vi "UI Coherent.vi"(8 "error in":errorcluster) -> (0 "error out":errorcluster)   [LabVIEW 2019, in "Coherent.lvlib"]
uses:
  Coherent.lvlib
  User Event/Controls/UE Abort Action.ctl
  <vilib>/Utility/miscctls.llb/LVPointTypeDef.ctl
  Queues/Queues.lvlib
panel:
  in  "Laser Control":T1={"Laser Switch"=FALSE, "Laser Power(mW)"=40} {"Laser Power(mW)" max=100}
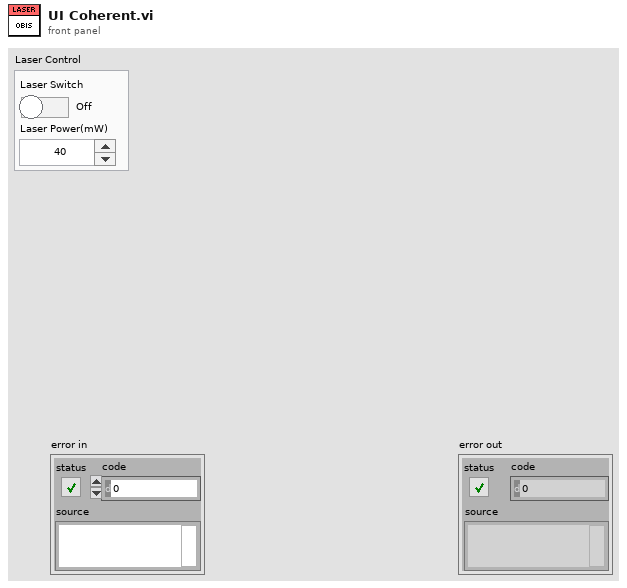
[diagram p1: front panel]
types:
  T1 = cluster{"Laser Switch":bool, "Laser Power(mW)":u16}
  T2 = typedef "UE Abort Action.ctl" = enum16{"Create", "Get", "Destroy"}
  T3 = enum16{"Start", "Get State", "On", "Off", "Set Power", "Change Mode", "Close"}
  T4 = typedef "LVPointTypeDef.ctl" = cluster{"Horizontal":i16, "Vertical":i16}
  T5 = typedef "Coherent.lvlib/SEQ Data.ctl" = cluster{"Initialize Success?":bool, "VI Refnum":refnum<vi>}
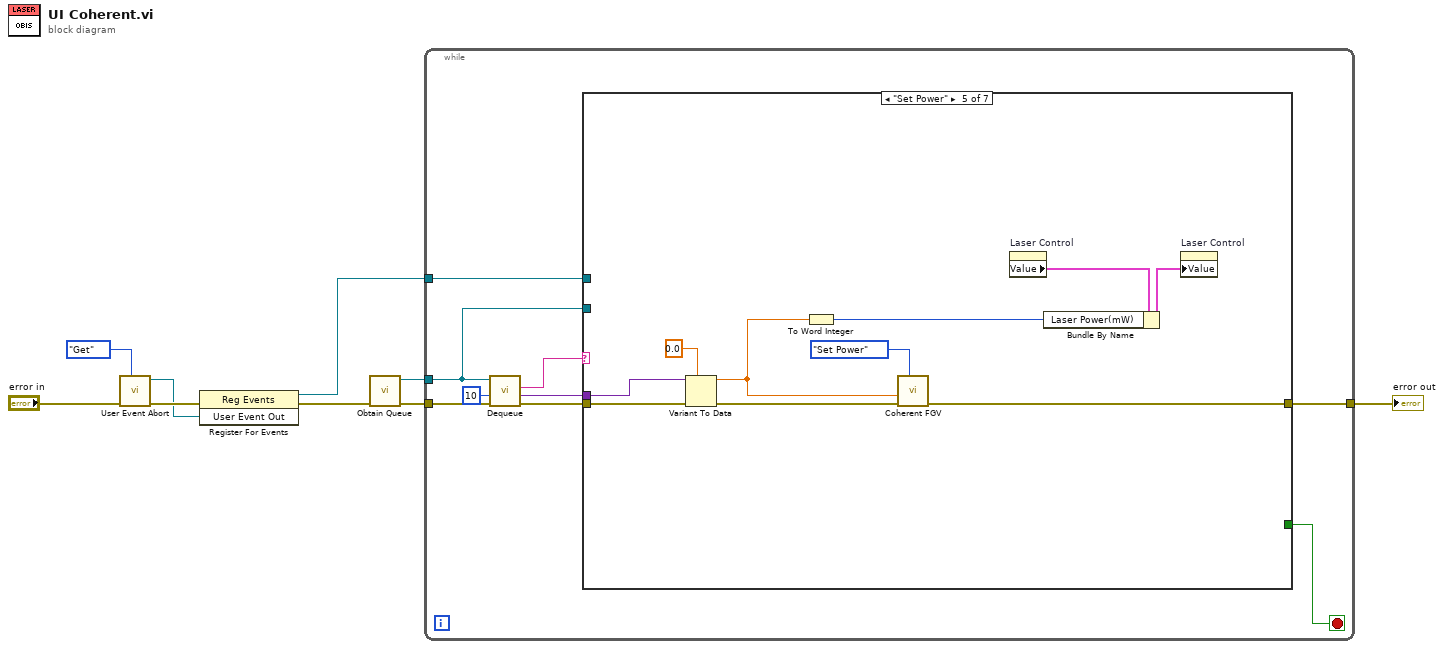
[diagram p0: block diagram]
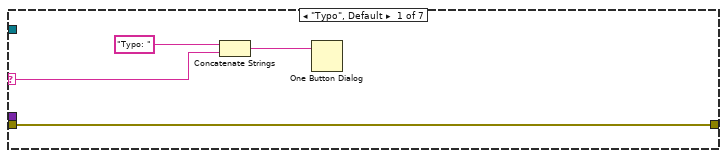
[diagram p2: hidden frame]
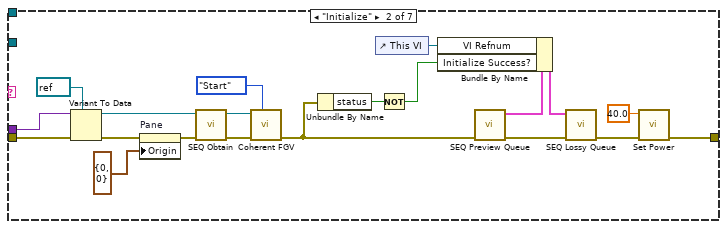
[diagram p3: hidden frame]
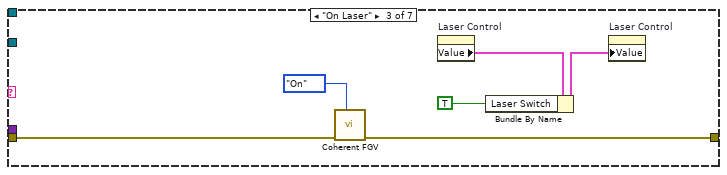
[diagram p4: hidden frame]
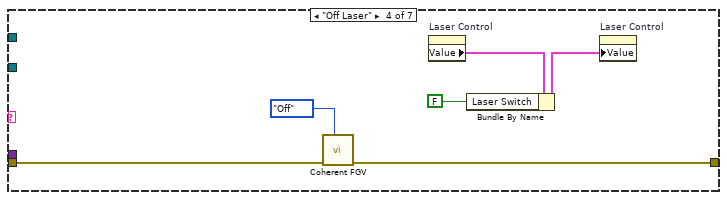
[diagram p5: hidden frame]
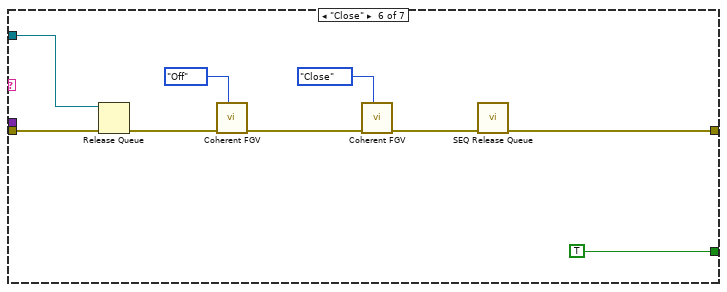
[diagram p6: hidden frame]
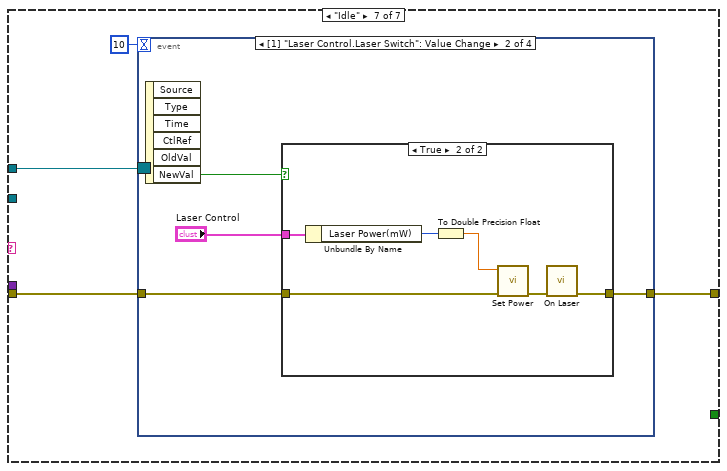
[diagram p7: hidden frame]
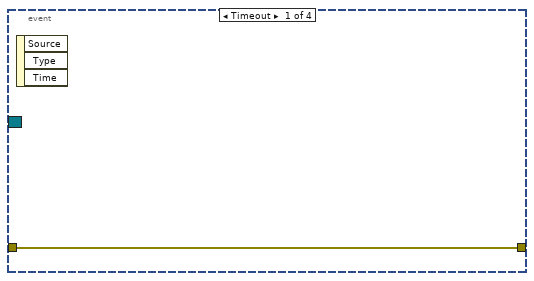
[diagram p8: hidden frame]
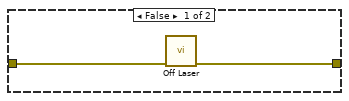
[diagram p9: hidden frame]
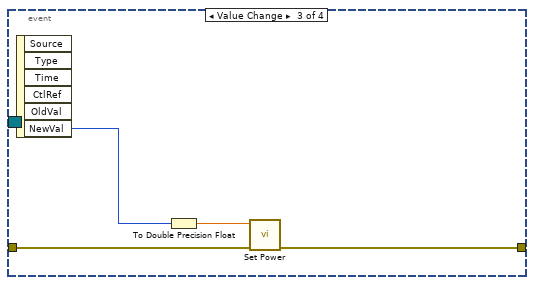
[diagram p10: hidden frame]
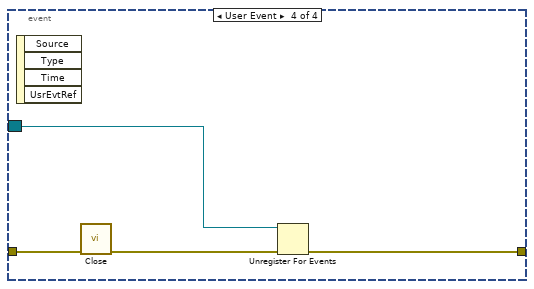
[diagram p11: hidden frame]
diagram:
  n1 = call "User Event Abort.vi"("Action"=UE_Abort_Action."Get", "Error In"="error in") -> ("Error Out"=w7:errorcluster, "User Event Out"=w6:refnum<user-event>)  [unwired: 8 in]
  n2 = register-events(error in=w7, w6) -> (reference out=w4:refnum<event-registration>, error out=w3:errorcluster)  [unwired: 1 in]
  n3 = call "Obtain Queue.vi"("Error In"=w3) -> ("Error Out"=w2:errorcluster, "Queue out"=w1:refnum<queue>)  [unwired: 9 in]
  n4 = while {
    tunnel: w2 -> [w18]
    tunnel: w1 -> [w13]
    tunnel: [w12] -> w5
    tunnel: w4 -> [w11]
    stop <- w10 stop-if-true
    n5 = call "Dequeue.vi"("Error In"=w18, "timeout in ms (-1)"=10, "Queue in"=w13) -> ("Error Out"=w17:errorcluster, "Data"=w15:variant, "State"=w16:string)  [unwired: 5 in, 1 out]
    n6 = case shown="\"Set Power\"" w16 {
      selector: w16 -> [w19 _ _ _ _ _ _]
      tunnel: w17 -> [w22 w29 w47 w53 w61 w72 w75]
      tunnel: w15 -> [_ w27 _ _ w59 _ _]
      tunnel: w13 -> [_ _ _ _ _ w71 _]
      tunnel: [w22 w39 w46 w52 w63 w67 w74] -> w12
      tunnel: w11 -> [_ _ _ _ _ _ w73]
      tunnel: [_ _ _ _ _ TRUE _] -> w10
      frame "Typo", Default {
        n7 = Concatenate Strings("Typo: " ("string"), w19) -> (w21:string)
        n8 = One Button Dialog(message=w21) -> ()  [unwired: 1 in, 1 out]
      }
      frame "Initialize" {
        n9 = Variant To Data(error in=w29, type=refnum<visa-resource-name> refnum ("VISA resource name in"), Variant=w27) -> (data=w25:refnum<visa-resource-name>, error out=w28:errorcluster)
        n10 = property on="Pane" class="Pane"(error in=w28, "Origin"=T4 {"Horizontal"=0, "Vertical"=0}) -> (error out=w40:errorcluster)  [unwired: 1 in, 1 out]
        n11 = call "SEQ Obtain.vi"("error in"=w40) -> ("error out"=w30:errorcluster)  [unwired: 9 in, 1 out]
        n12 = call "Coherent FGV.vi"("Funtion"=T3."Start", "error in"=w30, "VISA resource name in"=w25) -> ("error out"=w35:errorcluster)  [unwired: 7 in, 1 out]
        n13 = Unbundle By Name(w35) -> ("status"=w24:bool)
        n14 = control-ref of="This VI"() -> (w34:refnum<vi>)
        n15 = Not(x=w24) -> (.not. x?=w23:bool)
        n16 = call "SEQ Preview Queue.vi"("error in"=w35) -> ("error out"=w38:errorcluster, "SEQ Data"=w37:T5)  [unwired: 9 in]
        n17 = Bundle By Name(cluster=w37, "VI Refnum"=w34, "Initialize Success?"=w23) -> (w36:T5)
        n18 = call "SEQ Lossy Queue.vi"("error in"=w38, "SEQ Data"=w36) -> ("error out"=w32:errorcluster)  [unwired: 9 in]
        n19 = call "Set Power.vi"("Error In"=w32, "Power(mW)"=40.0) -> ("Error Out"=w39:errorcluster)  [unwired: 9 in]
      }
      frame "On Laser" {
        n20 = call "Coherent FGV.vi"("Funtion"=T3."On", "error in"=w47) -> ("error out"=w46:errorcluster)  [unwired: 8 in, 1 out]
        n21 = property on="Laser Control" class="Clust (strict)"() -> ("Value"=w44:T1)  [unwired: 2 in, 2 out]
        n22 = Bundle By Name(cluster=w44, "Laser Switch"=TRUE) -> (w43:T1)
        n23 = property on="Laser Control" class="Clust (strict)"("Value"=w43) -> ()  [unwired: 2 in, 2 out]
      }
      frame "Off Laser" {
        n24 = call "Coherent FGV.vi"("Funtion"=T3."Off", "error in"=w53) -> ("error out"=w52:errorcluster)  [unwired: 8 in, 1 out]
        n25 = property on="Laser Control" class="Clust (strict)"() -> ("Value"=w50:T1)  [unwired: 2 in, 2 out]
        n26 = Bundle By Name(cluster=w50, "Laser Switch"=FALSE) -> (w49:T1)
        n27 = property on="Laser Control" class="Clust (strict)"("Value"=w49) -> ()  [unwired: 2 in, 2 out]
      }
      frame "Set Power" {
        n28 = Variant To Data(error in=w61, type=0.0 ("Power(mW)"), Variant=w59) -> (data=w55:dbl, error out=w60:errorcluster)
        n29 = To Word Integer(number=w55) -> (16bit integer=w54:i16)
        n30 = call "Coherent FGV.vi"("Funtion"=T3."Set Power", "error in"=w60, "Power(mW)"=w55) -> ("error out"=w63:errorcluster)  [unwired: 7 in, 1 out]
        n31 = property on="Laser Control" class="Clust (strict)"() -> ("Value"=w57:T1)  [unwired: 2 in, 2 out]
        n32 = Bundle By Name(cluster=w57, "Laser Power(mW)"=w54) -> (w56:T1)
        n33 = property on="Laser Control" class="Clust (strict)"("Value"=w56) -> ()  [unwired: 2 in, 2 out]
      }
      frame "Close" {
        n34 = Release Queue(queue=w71, error in (no error)=w72) -> (error out=w65:errorcluster)  [unwired: 1 in, 2 out]
        n35 = call "Coherent FGV.vi"("Funtion"=T3."Off", "error in"=w65) -> ("error out"=w64:errorcluster)  [unwired: 8 in, 1 out]
        n36 = call "Coherent FGV.vi"("Funtion"=T3."Close", "error in"=w64) -> ("error out"=w68:errorcluster)  [unwired: 8 in, 1 out]
        n37 = call "SEQ Release Queue.vi"("error in"=w68) -> ("error out"=w67:errorcluster)  [unwired: 10 in]
      }
      frame "Idle" {
        n38 = event shown="[1] \"Laser Control.Laser Switch\": Value Change" {
          selector: w73 -> [_ _ _ w97]
          dyn-events: _ -> [_ _ _ _]
          timeout: 10 -> [_ _ _ _]
          tunnel: w75 -> [w77 w80 w93 w95]
          tunnel: [w77 w79 w92 w96] -> w74
          event Timeout {
            n39 = event-data() -> ()  [unwired: 1 in, 3 out]
          }
          event "Laser Control.Laser Switch": Value Change {
            n40 = event-data() -> ("NewVal"=w81:bool)  [unwired: 1 in, 5 out]
            n41 = case shown="True" w81 {
              tunnel: w80 -> [w83 w86]
              tunnel: [w82 w89] -> w79
              tunnel: "Laser Control" -> [_ w88]
              frame False {
                n42 = call "Off Laser.vi"("Error In"=w83) -> ("Error Out"=w82:errorcluster)  [unwired: 10 in]
              }
              frame True {
                n43 = Unbundle By Name(w88) -> ("Laser Power(mW)"=w87:u16)
                n44 = To Double Precision Float(number=w87) -> (double precision float=w84:dbl)
                n45 = call "Set Power.vi"("Error In"=w86, "Power(mW)"=w84) -> ("Error Out"=w85:errorcluster)  [unwired: 9 in]
                n46 = call "On Laser.vi"("Error In"=w85) -> ("Error Out"=w89:errorcluster)  [unwired: 10 in]
              }
            }
          }
          event "Laser Control.Laser Power(mW)": Value Change {
            n47 = event-data() -> ("NewVal"=w90:u16)  [unwired: 1 in, 5 out]
            n48 = To Double Precision Float(number=w90) -> (double precision float=w91:dbl)
            n49 = call "Set Power.vi"("Error In"=w93, "Power(mW)"=w91) -> ("Error Out"=w92:errorcluster)  [unwired: 9 in]
          }
          event User Event {
            n50 = event-data() -> ()  [unwired: 1 in, 4 out]
            n51 = call "Close.vi"("Error In"=w95) -> ("Error Out"=w94:errorcluster)  [unwired: 10 in]
            n52 = Unregister For Events(event registration refnum=w97, error in=w94) -> (error out=w96:errorcluster)
          }
        }
      }
    }
  }
  "error out" <- w5
